vi "FG VFH Queue.vi"(2 "FG Action":T1, 3 "VFH Queue in":refnum<queue>) -> (1 "VFH Queue out":refnum<queue>)   [LabVIEW 2009]
uses:
  Actions for FG's.ctl
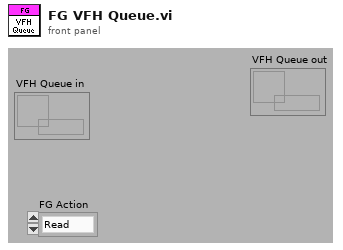
[diagram p1: front panel]
types:
  T1 = typedef "Actions for FG's.ctl" = enum16{"Read", "Write"}
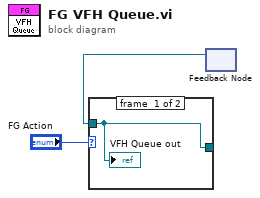
[diagram p0: block diagram]
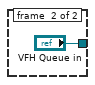
[diagram p2: hidden frame]
diagram:
  n1 = feedback #1() -> (w1:refnum<queue>)  [unwired: 1 in]
  n2 = case shown="\"Read\", Default" "FG Action" {
    tunnel: [w4 "VFH Queue in"] -> w2
    tunnel: w1 -> [w4 _]
    frame #0 {
      "VFH Queue out" <- w4
    }
    frame #1 {
    }
  }
